vi "4031Project.vi"() -> ()   [LabVIEW 2024]
uses:
  <vilib>/Utility/file.llb/Write Delimited Spreadsheet (string).vi
  <vilib>/Utility/TradDaqScaling.llb/Convert Thermocouple Reading (array).vi
  <vilib>/Utility/file.llb/Write Delimited Spreadsheet (DBL).vi
  <vilib>/Analysis/NI_AALBase.lvlib
panel:
  out "Tco Std":dbl
  out "Tco Mean":dbl
  out "Waveform Chart 4":sgl[](graph)
  in  "ThermocoupleType 4":u16(ring)=2 items=["B", "E", "J", "K", "R", "S", "T", "N"]
  out "Tci Std":dbl
  out "Tci Mean":dbl
  out "Waveform Chart 3":sgl[](graph)
  in  "ThermocoupleType 3":u16(ring)=2 items=["B", "E", "J", "K", "R", "S", "T", "N"]
  out "Tho SD 2":dbl
  out "Tho mean":dbl
  out "Waveform Chart 2":sgl[](graph)
  in  "ThermocoupleType 2":u16(ring)=2 items=["B", "E", "J", "K", "R", "S", "T", "N"]
  out "Thi SD":dbl
  out "Thi mean":dbl
  out "Waveform Chart":sgl[](graph)
  in  "ThermocoupleType":u16(ring)=2 items=["B", "E", "J", "K", "R", "S", "T", "N"]
  in  "stop":bool
  in  "Sampling rate":dbl
  in  "Number of Samples":dbl
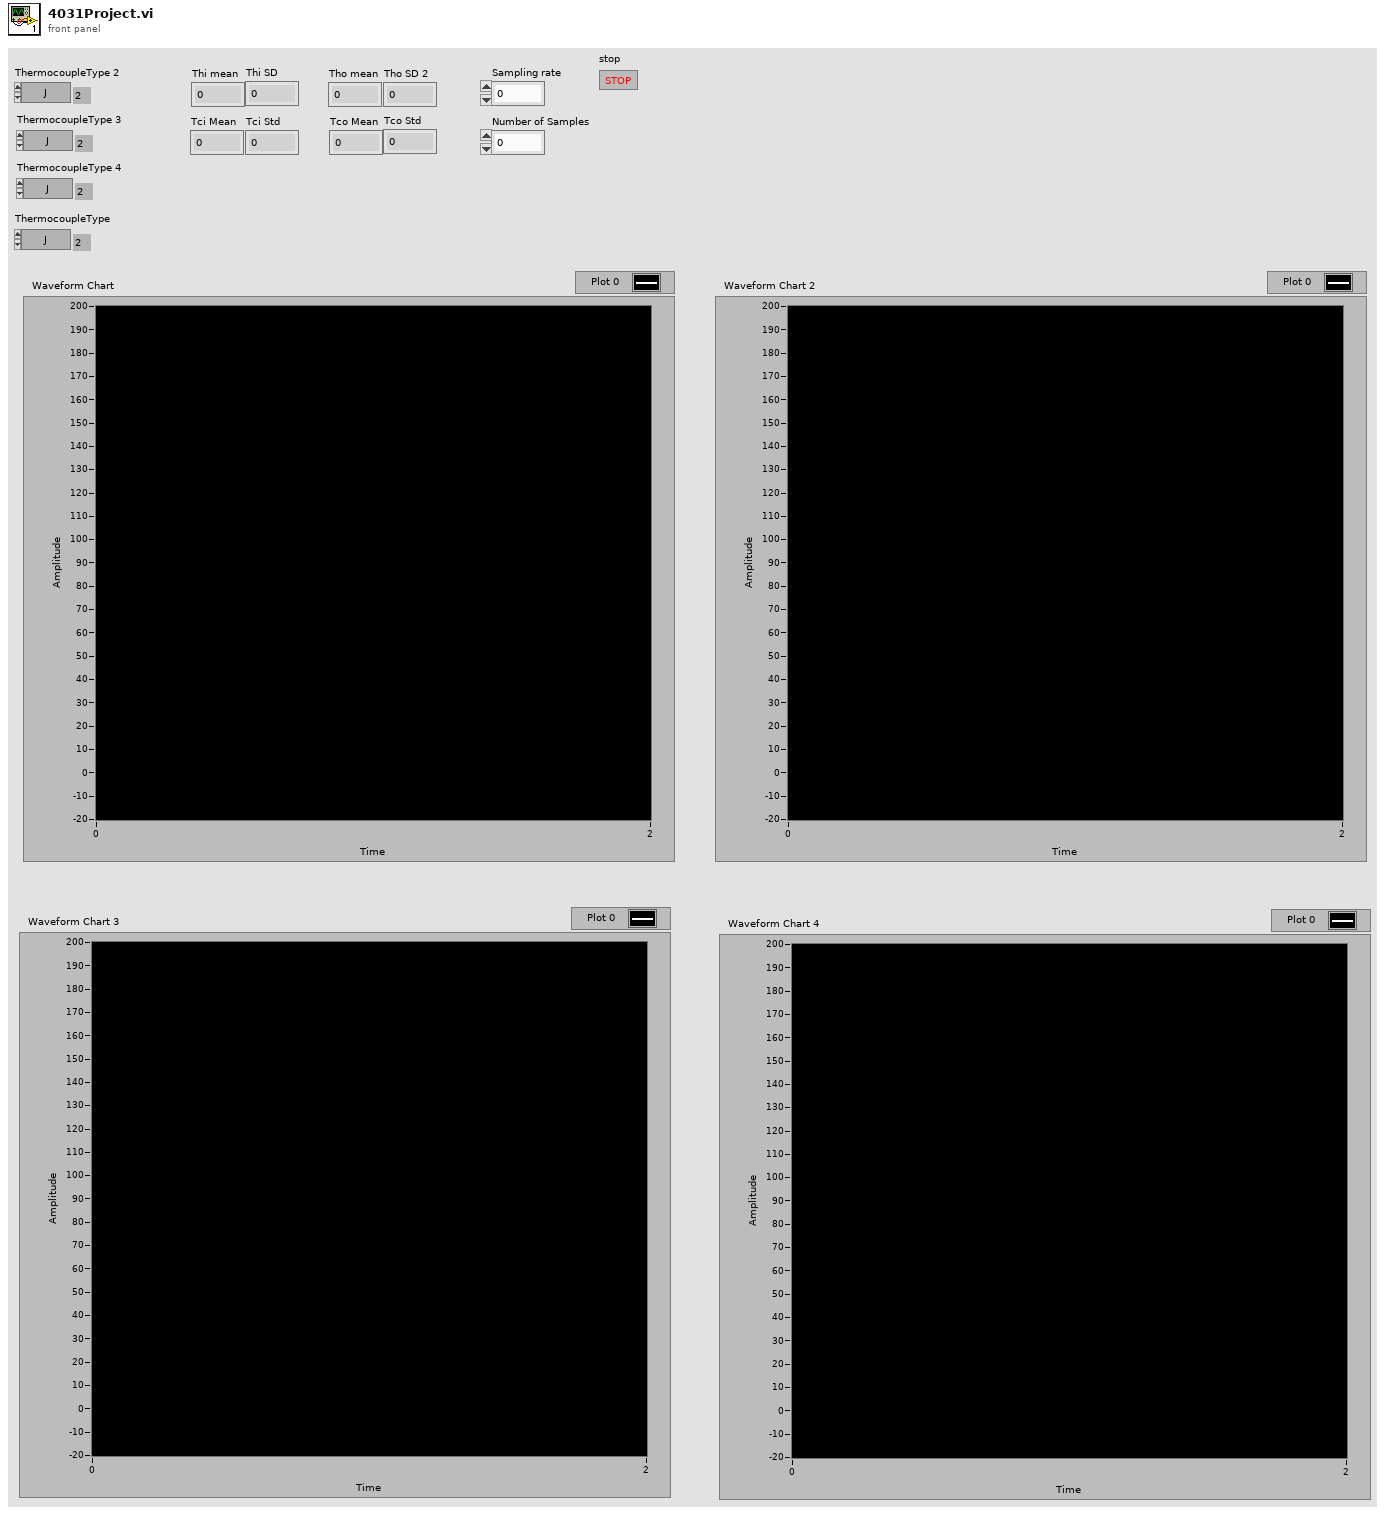
[diagram p1: front panel]
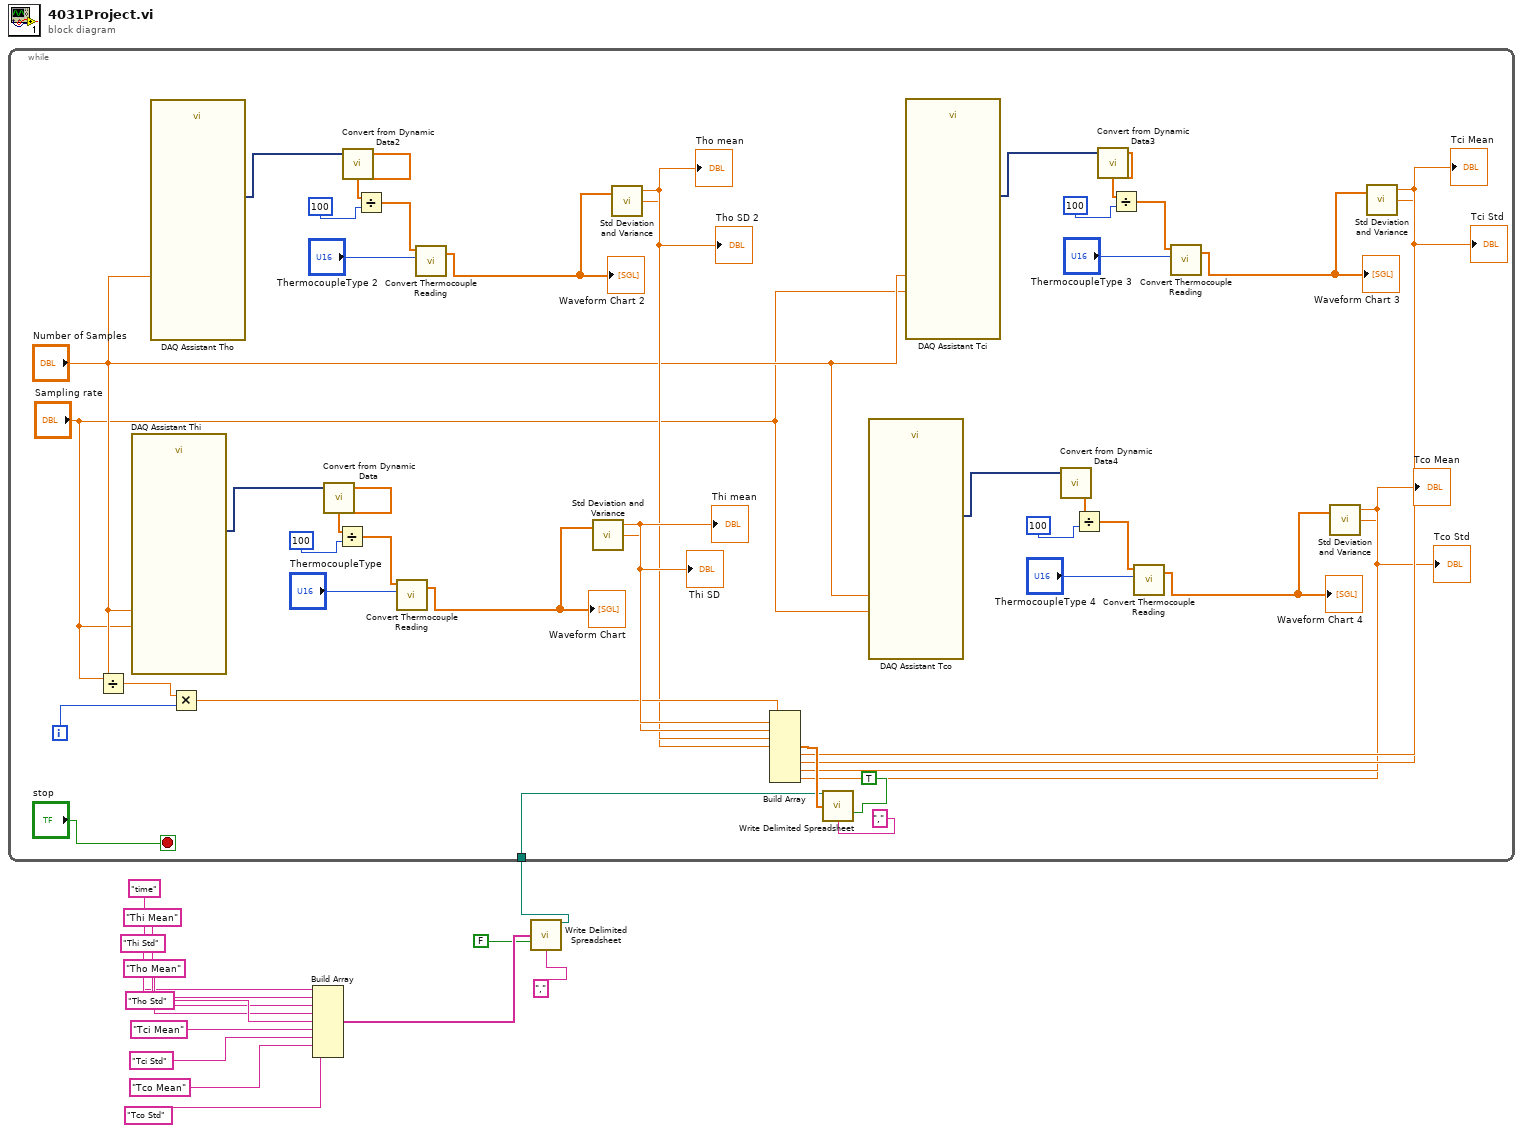
[diagram p0: block diagram]
diagram:
  n1 = Build Array("time", "Thi Mean", "Thi Std", "Tho Mean", "Tho Std", "Tci Mean", "Tci Std", "Tco Mean", "Tco Std") -> (w9:string[])
  n2 = call-poly <vilib>:"Write Delimited Spreadsheet.vi"("1D data"=w9, "append to file? (new file:F)"=FALSE, "delimiter (\\t)"=",") -> ("new file path (Not A Path if cancelled)"=w7:path)  [unwired: 11 in, 1 out]
  n3 = while {
    tunnel: w7 -> [w50]
    i -> [w29]
    stop <- "stop" stop-if-true
    n4 = Divide(x="Sampling rate", y="Number of Samples") -> (x/y=w45:dbl)
    n5 = call "DAQ Assistant Thi"("rate"="Sampling rate", "number of samples"="Number of Samples") -> ("data"=w44:dynamicdata)  [unwired: 15 in, 2 out]
    n6 = call "DAQ Assistant Tho"("number of samples"="Number of Samples") -> ("data"=w38:dynamicdata)  [unwired: 16 in, 2 out]
    n7 = Multiply(x=w45, y=w29) -> (x*y=w22:dbl)
    n8 = call "Convert from Dynamic Data"("Dynamic Data Type"=w44) -> ("Array"=w48:dbl[])  [unwired: 3 in]
    n9 = Divide(x=w48, y=100) -> (x/y=w47:dbl[])
    n10 = call "Convert from Dynamic Data2"("Dynamic Data Type"=w38) -> ("Array"=w41:dbl[])  [unwired: 3 in]
    n11 = Divide(x=w41, y=100) -> (x/y=w40:dbl[])
    n12 = call-poly <vilib>:"Convert Thermocouple Reading.vi"("ThermocoupleType"="ThermocoupleType", "Voltage Array"=w47) -> ("Temperature Array"=w46:sgl[])  [unwired: 5 in]
    "Waveform Chart" <- w46
    n13 = call-poly <vilib>:"Convert Thermocouple Reading.vi"("ThermocoupleType"="ThermocoupleType 2", "Voltage Array"=w40) -> ("Temperature Array"=w39:sgl[])  [unwired: 5 in]
    "Waveform Chart 2" <- w39
    n14 = call <vilib>:"Std Deviation and Variance.vi"("X"=w46) -> ("mean"=w24:dbl, "standard deviation"=w23:dbl)  [unwired: 1 in, 1 out]
    "Thi mean" <- w24
    "Thi SD" <- w23
    n15 = call <vilib>:"Std Deviation and Variance.vi"("X"=w39) -> ("mean"=w21:dbl, "standard deviation"=w20:dbl)  [unwired: 1 in, 1 out]
    "Tho mean" <- w21
    "Tho SD 2" <- w20
    n16 = call "DAQ Assistant Tco"("rate"="Sampling rate", "number of samples"="Number of Samples") -> ("data"=w26:dynamicdata)  [unwired: 15 in, 2 out]
    n17 = call "DAQ Assistant Tci"("rate"="Sampling rate", "number of samples"="Number of Samples") -> ("data"=w28:dynamicdata)  [unwired: 15 in, 2 out]
    n18 = call "Convert from Dynamic Data4"("Dynamic Data Type"=w26) -> ("Array"=w25:dbl[])  [unwired: 3 in]
    n19 = Divide(x=w25, y=100) -> (x/y=w31:dbl[])
    n20 = call "Convert from Dynamic Data3"("Dynamic Data Type"=w28) -> ("Array"=w27:dbl[])  [unwired: 3 in]
    n21 = Divide(x=w27, y=100) -> (x/y=w35:dbl[])
    n22 = call-poly <vilib>:"Convert Thermocouple Reading.vi"("ThermocoupleType"="ThermocoupleType 4", "Voltage Array"=w31) -> ("Temperature Array"=w30:sgl[])  [unwired: 5 in]
    "Waveform Chart 4" <- w30
    n23 = call-poly <vilib>:"Convert Thermocouple Reading.vi"("ThermocoupleType"="ThermocoupleType 3", "Voltage Array"=w35) -> ("Temperature Array"=w34:sgl[])  [unwired: 5 in]
    "Waveform Chart 3" <- w34
    n24 = call <vilib>:"Std Deviation and Variance.vi"("X"=w30) -> ("mean"=w17:dbl, "standard deviation"=w16:dbl)  [unwired: 1 in, 1 out]
    "Tco Mean" <- w17
    "Tco Std" <- w16
    n25 = call <vilib>:"Std Deviation and Variance.vi"("X"=w34) -> ("mean"=w19:dbl, "standard deviation"=w18:dbl)  [unwired: 1 in, 1 out]
    "Tci Mean" <- w19
    "Tci Std" <- w18
    n26 = Build Array(w22, w24, w23, w21, w20, w19, w18, w17, w16) -> (w52:dbl[])
    n27 = call-poly <vilib>:"Write Delimited Spreadsheet.vi"("file path (dialog if empty)"=w50, "1D data"=w52, "append to file? (new file:F)"=TRUE, "delimiter (\\t)"=",") -> ()  [unwired: 10 in, 2 out]
  }
